vi "AttackerAimGoalSkill.vi"(6 "AttackOurselves":bool, 8 "error in (no error)":errorcluster, 9 "Game":refnum<class "Game.lvclass">, 10 "Robot":refnum<class "Robot.lvclass">, 11 "AttackerAimGoalSkill in":refnum<class "AttackerAimGoalSkill.lvclass">) -> (0 "error out":errorcluster, 2 "Robot out":refnum<class "Robot.lvclass">, 3 "AttackerAimGoalSkill out":refnum<class "AttackerAimGoalSkill.lvclass">)   [LabVIEW 2018, in "AttackerAimGoalSkill.lvclass"]
uses:
  AttackerAimGoalSkill.lvclass
  Robot_class/Robot.lvclass
  C:/Users/nicolas.oliveira/roboime/SSL_AI/Object_class/Object.lvclass
  Game_class/Game.lvclass
  Utilities_class/Utilities.lvclass
  Game_class/Game.lvclass/Game.ctl
  Parameters_class/Parameters.lvclass/Parameters.ctl
  Object_class/Object.lvclass/Object.ctl
  Robot_class/Robot.lvclass/Robot.ctl
  <vilib>/Analysis/_algsub.llb/Real Vector Norm.vi
  Game_class/Read Parameters.lvclass.vi
  Parameters_class/Read DistanceStop.vi
  Game_class/Read BallRef.vi
  Game_class/Read FieldRef.vi
  Object_class/Read x.vi
  Object_class/Read y.vi
  Robot_class/Write dest_x.vi
  Robot_class/Write dest_y.vi
  Robot_class/Write dest_orientation.vi
  Robot_class/Write dest_x_kick.vi
  Robot_class/Write dest_y_kick.vi
  Ball_class/Ball.lvclass
  Field_class/Field.lvclass
  Parameters_class/Parameters.lvclass
  <vilib>/Analysis/NI_AALPro.lvlib
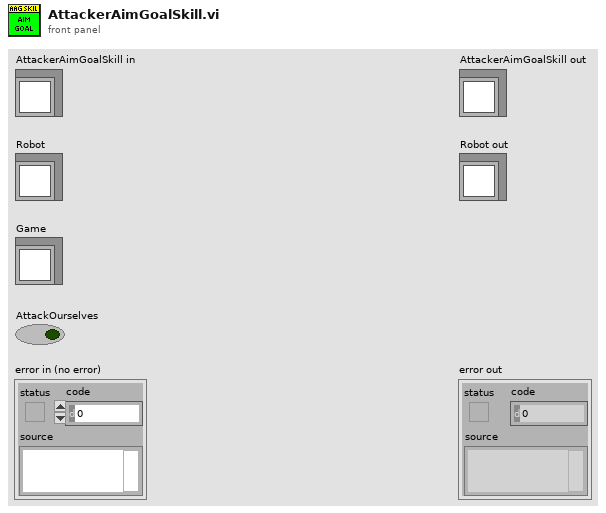
[diagram p1: front panel]
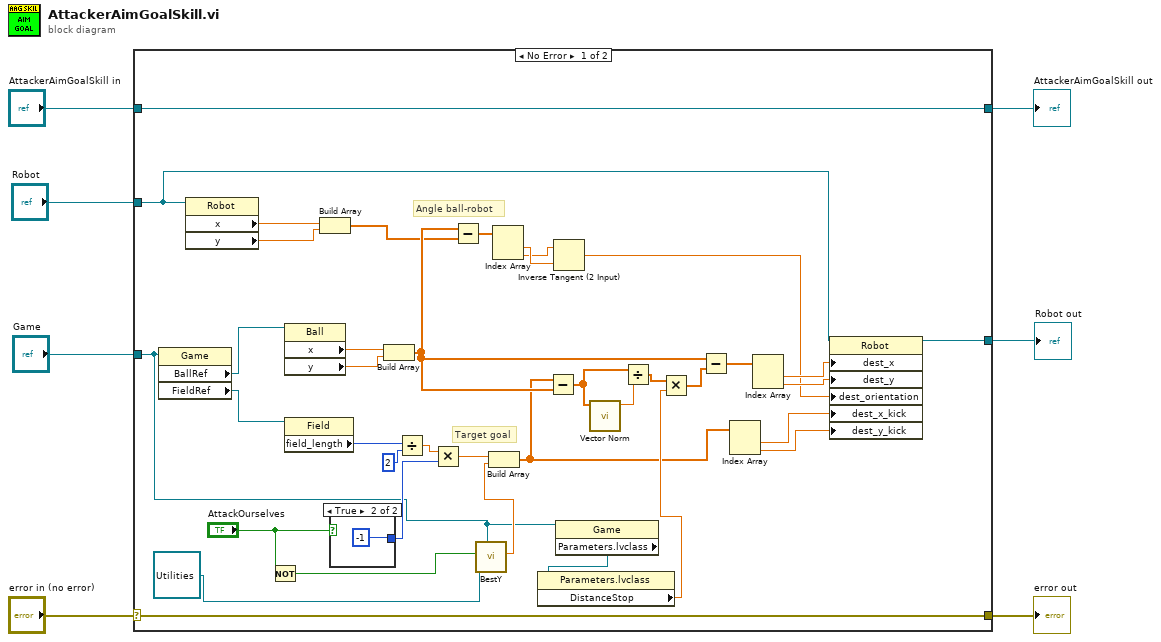
[diagram p0: block diagram]
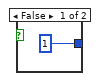
[diagram p2: hidden frame]
diagram:
  n1 = case shown="No Error" "error in (no error)" {
    selector: "error in (no error)" -> [w44 w50]
    tunnel: [w44 w50] -> w6
    tunnel: [w45 w49] -> w4
    tunnel: "AttackerAimGoalSkill in" -> [w45 w49]
    tunnel: "Robot" -> [w18 w48]
    tunnel: "Game" -> [w13 _]
    tunnel: [w14 w48] -> w1
    frame No Error {
      # "Angle ball-robot"
      # "Target goal"
      n2 = property class="Game"(reference=w13) -> ("BallRef"=w43:refnum<class "Ball.lvclass">, "FieldRef"=w42:refnum<class "Field.lvclass">)  [unwired: 1 in, 2 out]
      n3 = property class="Robot"(reference=w18) -> ("x"=w26:dbl, "y"=w25:dbl)  [unwired: 1 in, 2 out]
      n4 = Not(x="AttackOurselves") -> (.not. x?=w27:bool)
      n5 = property class="Ball"(reference=w43) -> ("x"=w36:dbl, "y"=w35:dbl)  [unwired: 1 in, 2 out]
      n6 = property class="Field"(reference=w42) -> ("field_length"=w41:i32)  [unwired: 1 in, 2 out]
      n7 = Build Array(w26, w25) -> (w23:dbl[])
      n8 = case shown="True" "AttackOurselves" {
        tunnel: [1 -1] -> w38
        frame False {
        }
        frame True {
        }
      }
      n9 = Build Array(w36, w35) -> (w24:dbl[])
      n10 = Divide(x=w41, y=2) -> (x/y=w39:dbl)
      n11 = Multiply(x=w39, y=w38) -> (x*y=w37:dbl)
      n12 = Subtract(x=w24, y=w23) -> (x-y=w22:dbl[])
      n13 = call-dynamic "BestY.vi"("Game"=w13, "inimigos"=w27, "Utilities in"=refnum<class "Utilities.lvclass"> refnum) -> ("Best y"=w30:dbl)  [unwired: 3 in, 5 out]
      n14 = Build Array(w37, w30) -> (w10:dbl[])
      n15 = Index Array(array=w22) -> (element #1=w21:dbl, element #2=w20:dbl)  [unwired: 2 in]
      n16 = Subtract(x=w10, y=w24) -> (x-y=w34:dbl[])
      n17 = Inverse Tangent (2 Input)(1:w21, 2:w20) -> (0:w15:dbl)
      n18 = property class="Game"(reference=w13) -> ("Parameters.lvclass"=w12:refnum<class "Parameters.lvclass">)  [unwired: 1 in, 2 out]
      n19 = property class="Parameters.lvclass"(reference=w12) -> ("DistanceStop"=w11:dbl)  [unwired: 1 in, 2 out]
      n20 = call-poly <vilib>:"Vector Norm.vi"("Input Vector"=w34) -> ("norm"=w33:dbl)  [unwired: 9 in, 1 out]
      n21 = Divide(x=w34, y=w33) -> (x/y=w32:dbl[])
      n22 = Multiply(x=w32, y=w11) -> (x*y=w31:dbl[])
      n23 = Subtract(x=w24, y=w31) -> (x-y=w19:dbl[])
      n24 = Index Array(array=w10) -> (element #1=w9:dbl, element #2=w8:dbl)  [unwired: 2 in]
      n25 = Index Array(array=w19) -> (element #1=w17:dbl, element #2=w16:dbl)  [unwired: 2 in]
      n26 = property class="Robot"(reference=w18, "dest_x"=w17, "dest_y"=w16, "dest_orientation"=w15, "dest_x_kick"=w9, "dest_y_kick"=w8) -> (reference out=w14:refnum<class "Robot.lvclass">)  [unwired: 1 in, 1 out]
    }
    frame Error {
    }
  }
  "error out" <- w6
  "AttackerAimGoalSkill out" <- w4
  "Robot out" <- w1
